vi "saltso prueba.vi"() -> ()   [LabVIEW 2010]
uses:
  <vilib>/vision/Image Controls.llb/IMAQ Image.ctl
panel:
  in  "Numero Ultimo Experimento":i32
  out "Tomando Saltos":bool=TRUE
  out "Estable":bool=TRUE
  in  "Path":path
  out "appended path":path
  out "Freq Output":dbl
  in  "Image Device IN":cluster{"Image":T1, "errorImage":errorcluster}
  in  "Comienza Saltos":bool=TRUE
  in  "Parametros de Saltos":T2
  in  "stop":bool
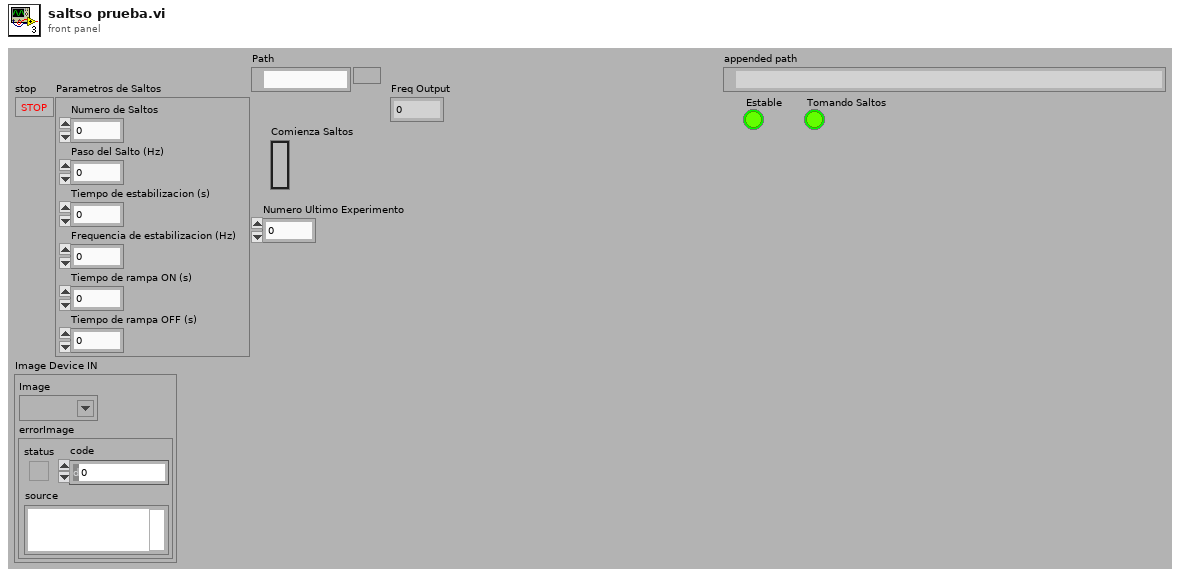
[diagram p1: front panel]
types:
  T1 = typedef "IMAQ Image.ctl" = refnum<image>
  T2 = cluster{"Numero de Saltos":i32, "Paso del Salto (Hz)":dbl, "Tiempo de estabilizacion (s)":dbl, "Frequencia de estabilizacion (Hz)":dbl, "Tiempo de rampa ON (s)":dbl, "Tiempo de rampa OFF (s)":dbl}
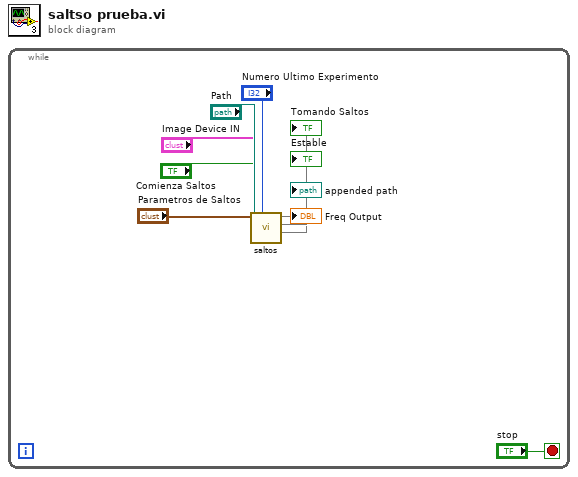
[diagram p0: block diagram]
diagram:
  n1 = while {
    stop <- "stop" stop-if-true
    n2 = call "saltos.vi"(4:"Numero Ultimo Experimento", 5:"Image Device IN", 6:"Comienza Saltos", 7:"Path", 8:"Parametros de Saltos") -> (0:→"Tomando Saltos", 1:→"Estable", 2:→"appended path", 3:→"Freq Output")
  }
